vi "GEA2 Serial Dryer Command Needs Read.vi"(5 "Command 2":T1 items=["CMD_Eval_Mode_Entry_CC1", "CMD_Eval_Mode_Entry_CC2", "CMD_Eval_Mode_Continue", "CMD_Send_DIAG_Info", "CMD_Enable_Debug_Log ", "CMD_Disable_Debug_Log ", "CMD_Send_Log_Data", "CMD_Stop", "RQST_Version"], 11 "Error In":errorcluster) -> (6 "RQST":bool, 15 "Error Out":errorcluster)   [LabVIEW 2014]
uses:
  Type Definitions/GEA2 Serial Dryer Commands.ctl
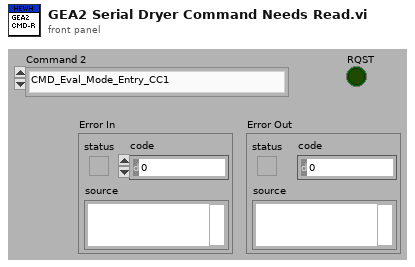
[diagram p1: front panel]
types:
  T1 = typedef "GEA2 Serial Dryer Commands.ctl" = u8
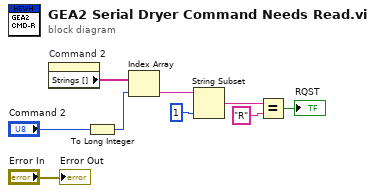
[diagram p0: block diagram]
diagram:
  n1 = property on="Command 2" class="Ring (strict)"() -> ("Strings []"=w2:string[])  [unwired: 2 in, 2 out]
  n2 = To Long Integer(number="Command 2") -> (32bit integer=w8:i32)
  n3 = Index Array(array=w2, index=w8) -> (element=w7:string)
  n4 = String Subset(string=w7, length (rest)=1 ("length (rest)")) -> (substring=w5:string)  [unwired: 1 in]
  n5 = Equal?(x=w5, y="R") -> (x = y?=→"RQST":bool)
  "Error Out" <- "Error In"
